vi "GenKnightRider.vi"(5 "Background Color":u32(colorbox), 6 "Reset":bool, 7 "Foreground Color":u32(colorbox)=16711680, 9 "Blending LEDs":u8=10, 10 "Sine Rate":i32, 11 "NumLeds":i32) -> (2 "Iterations":i32, 3 "Array":u32[](array[numeric]))   [LabVIEW 2020, in "ArduinoSerialBling.lvlib"]
uses:
  ArduinoSerialBling.lvlib
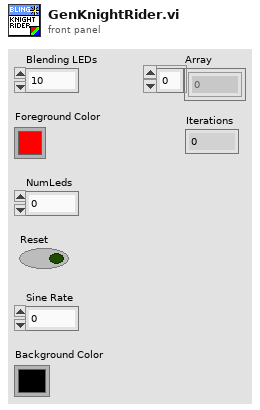
[diagram p1: front panel]
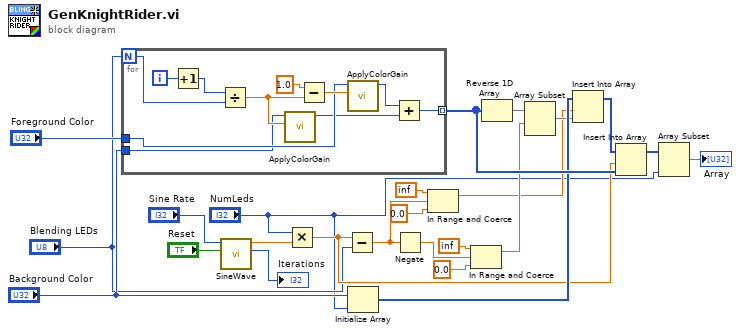
[diagram p0: block diagram]
diagram:
  n1 = for {
    N: "Blending LEDs" -> [w34]
    tunnel: "Foreground Color" -> [w28]
    tunnel: [w31] -> w17 mode=indexing
    tunnel: "Background Color" -> [w27]
    i -> [w35]
    n2 = Increment(x=w35) -> (x+1=w33:i32)
    n3 = Divide(x=w33, y=w34) -> (x/y=w30:dbl)
    n4 = call "ApplyColorGain.vi"("Gain"=w30, "Color In"=w27) -> ("Color Out"=w26:u32)  [unwired: 9 in]
    n5 = Subtract(x=1.0, y=w30) -> (x-y=w29:dbl)
    n6 = call "ApplyColorGain.vi"("Gain"=w29, "Color In"=w28) -> ("Color Out"=w25:u32)  [unwired: 9 in]
    n7 = Add(x=w25, y=w26) -> (x+y=w31:u32)
  }
  n8 = call "SineWave.vi"("Reset"="Reset", "Sine Rate"="Sine Rate") -> ("Iterator"=→"Iterations":i32, "Value (0-1)"=w14:dbl)  [unwired: 8 in]
  n9 = Multiply(x="NumLeds", y=w14) -> (x*y=w13:dbl)
  n10 = Subtract(x=w13, y="Blending LEDs") -> (x-y=w3:dbl)
  n11 = Initialize Array("Background Color", "NumLeds") -> (w16:u32[])
  n12 = Negate(x=w3) -> (-x=w9:dbl)
  n13 = In Range and Coerce(upper limit=inf, x=w3, lower limit=0.0) -> (coerced(x)=w2:dbl)  [unwired: 1 out]
  n14 = In Range and Coerce(upper limit=inf, x=w9, lower limit=0.0) -> (coerced(x)=w7:dbl)  [unwired: 1 out]
  n15 = Reverse 1D Array(array=w17) -> (reversed array=w11:u32[])
  n16 = Array Subset(array=w11, index=w7) -> (w10:u32[])  [unwired: 1 in]
  n17 = Insert Into Array(array=w16, index=w2, new element=w10) -> (w18:u32[])
  n18 = Insert Into Array(array=w18, index=w13, new element=w17) -> (w15:u32[])
  n19 = Array Subset(array=w15, length="NumLeds") -> (→"Array":u32[])  [unwired: 1 in]
